vi "Piston Solenoid.vi"(10 "Value":T4, 11 "Enum":enum16{"Start", "Run", "End"}(ring)=enum."Run") -> ()   [LabVIEW 2012]
uses:
  <vilib>/Rock Robotics/WPI/Solenoid/WPI_SolenoidValue.ctl
  TypeDefs/Solenoid Module 1.ctl
  <vilib>/Rock Robotics/WPI/Solenoid/WPI_SolenoidChannel.ctl
  <vilib>/Rock Robotics/SystemInterfaces/Typedef/FPGA_TypedefSolenoidModule.ctl
  <vilib>/Rock Robotics/WPI/Solenoid/WPI_SolenoidOpenDouble.vi
  <vilib>/Rock Robotics/WPI/Solenoid/WPI_SolenoidSetEnum.vi
panel:
  in  "Solenoid Module 1":T1={"Shoot FWD"=enum."Solenoid 1", "Shoot REV"=enum."Solenoid 2", "Climber"=enum."Solenoid 3", "Climber"=enum."Solenoid 4", "Arm Lock"=enum."Solenoid 5", "Unassigned"=enum."Solenoid 6", "Color"=enum."Solenoid 7", "Unassigned"=enum."Solenoid 8", "Module"=enum."Solenoid Module 1"}
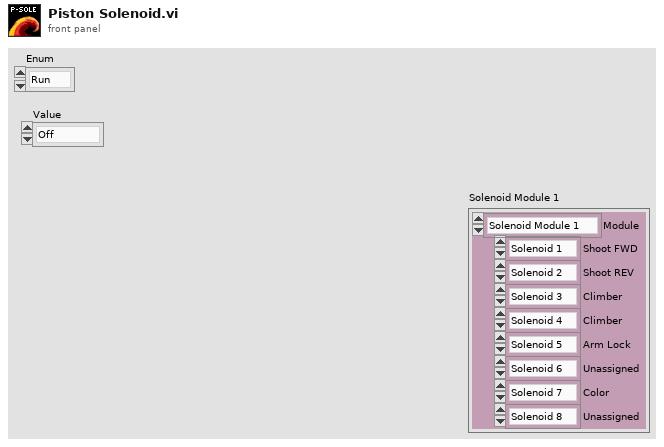
[diagram p1: front panel]
types:
  T1 = typedef "Solenoid Module 1.ctl" = cluster{"Shoot FWD":T2, "Shoot REV":T2, "Climber":T2, "Climber":T2, "Arm Lock":T2, "Unassigned":T2, "Color":T2, "Unassigned":T2, "Module":T3}
  T2 = typedef "WPI_SolenoidChannel.ctl" = enum8{"Solenoid 1", "Solenoid 2", "Solenoid 3", "Solenoid 4", "Solenoid 5", "Solenoid 6", "Solenoid 7", "Solenoid 8", "Invalid"}
  T3 = typedef "FPGA_TypedefSolenoidModule.ctl" = enum16{"Solenoid Module 1", "Solenoid Module 2"}
  T4 = typedef "WPI_SolenoidValue.ctl" = enum16{"Off", "On", "Forward", "Reverse"}
  T5 = typedef "WPI_SolenoidDevRef.ctl" = cluster{"DevStatus":errorcluster, "Solenoid Module":T3, "Forward Solenoid Channel":T2, "Reverse Solenoid Channel":T2}
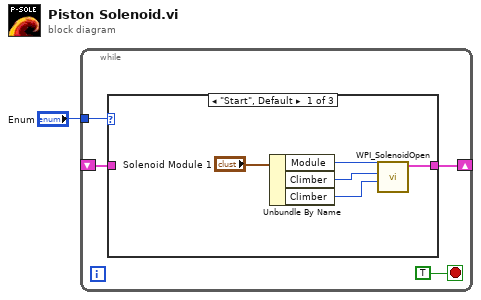
[diagram p0: block diagram]
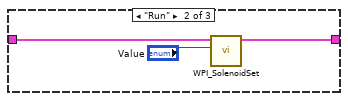
[diagram p2: hidden frame]
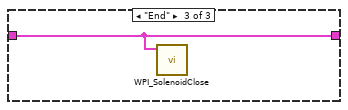
[diagram p3: hidden frame]
diagram:
  n1 = while {
    shift-right: [w5] -> _
    shift-left: _ -> [w3]
    tunnel: "Enum" -> [w4]
    stop <- TRUE stop-if-true
    n2 = case shown="\"Start\", Default" w4 {
      tunnel: [w10 w13 w14] -> w5
      tunnel: w3 -> [_ w12 w14]
      frame "Start", Default {
        n3 = Unbundle By Name("Solenoid Module 1") -> ("Module"=w8:T3, "Climber"=w7:T2, "Climber"=w6:T2)
        n4 = call-poly <vilib>:"WPI_SolenoidOpen.vi"("Reverse Solenoid Channel"=w6, "Forward Solenoid Channel"=w7, "Solenoid Module (Module 1)"=w8) -> ("SolenoidDevRef"=w10:T5)  [unwired: 7 in, 1 out]
      }
      frame "Run" {
        n5 = call-poly <vilib>:"WPI_SolenoidSet.vi"("Value"="Value", "SolenoidDevRef"=w12) -> ("SolenoidDevRef"=w13:T5)  [unwired: 8 in, 1 out]
      }
      frame "End" {
        n6 = call <vilib>:"WPI_SolenoidClose.vi"("SolenoidDevRef"=w14) -> ()  [unwired: 10 in, 1 out]
      }
    }
  }
